vi "Parse State Queue__JKI_lib_State_Machine_ACBMOD.vi"(0 "State Queue":string, 7 "Error In":errorcluster) -> (4 "Remaining States":string, 6 "Current State":string, 8 "Arguments":string)   [LabVIEW 2015]
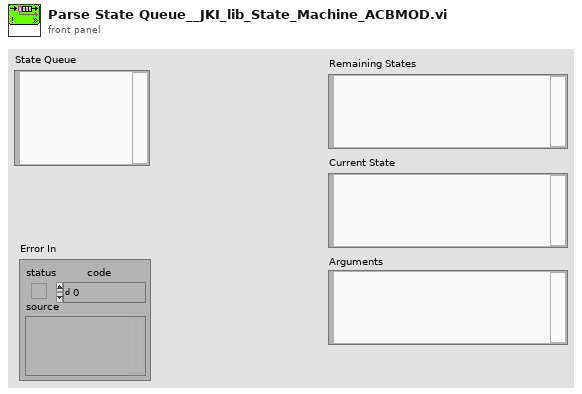
[diagram p1: front panel]
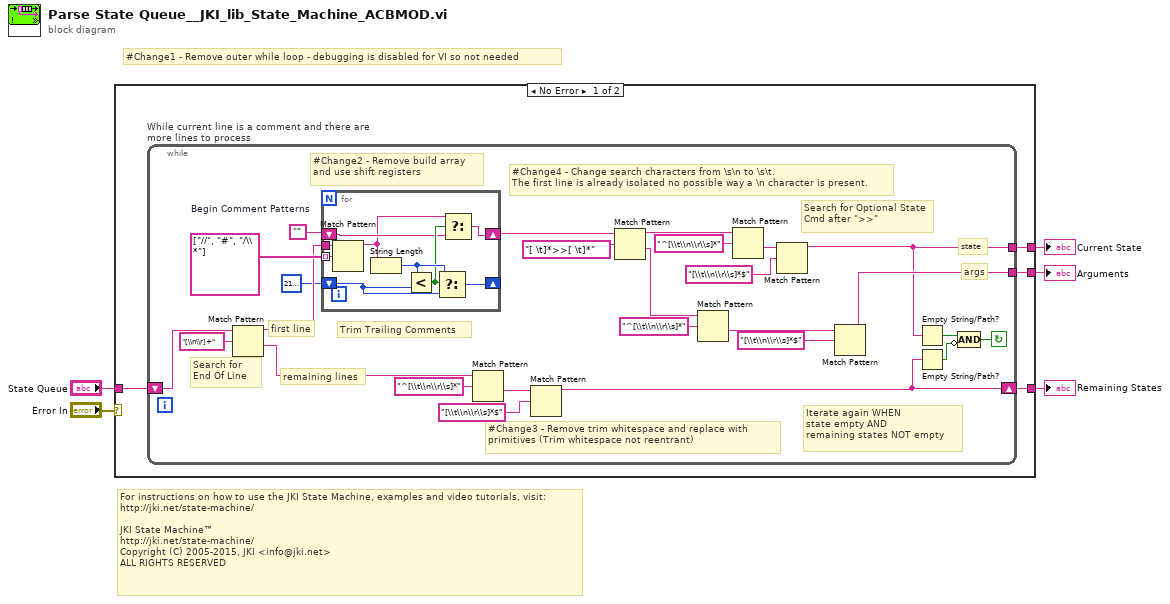
[diagram p0: block diagram]
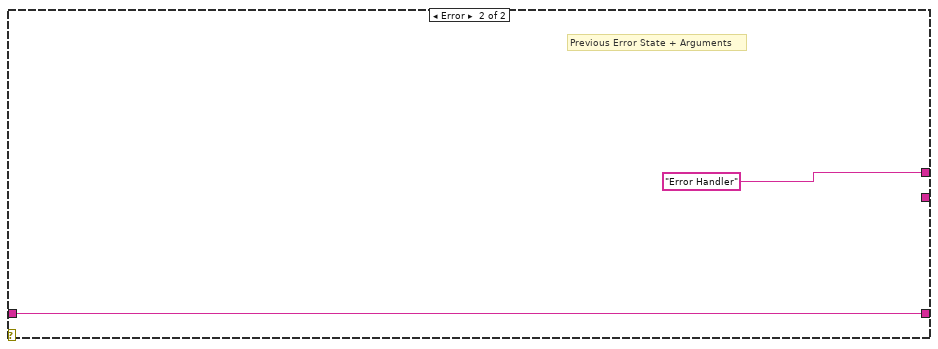
[diagram p2: hidden frame]
diagram:
  # "#Change1 - Remove outer while loop - debugging is disabled for VI so not needed"
  # "For instructions on how to use the JKI State Machine, examples and video tutorials, visit:\nhttp://jki.net/state-machine/\n\nJKI State Machine™\nhttp://jki.net/state-machine/\nCopyright (C) 2005-2015, JKI <info@jki.net>\nALL RIGHTS RESERVED"
  n1 = case shown="No Error" "Error In" {
    tunnel: [w6 w46] -> w5
    tunnel: [w9 "Error Handler"] -> w2
    tunnel: [w8 _] -> w1
    tunnel: "State Queue" -> [w7 w46]
    frame No Error {
      n2 = while "While current line is a comment and there are more lines to process" {
        tunnel: [w13] -> w9
        tunnel: [w21] -> w8
        shift-right: [w23] -> w6
        shift-left: w7 -> [w29]
        stop <- w31 continue-if-true
        w35 = string[] ["//", "#", "/\\*"]  # Begin Comment Patterns
        # "#Change4 - Change search characters from \\s\\n to \\s\\t.\nThe first line is already isolated no possible way a \\n character is present."
        # "#Change3 - Remove trim whitespace and replace with primitives (Trim whitespace not reentrant)"
        # "#Change2 - Remove build array and use shift registers"
        # "remaining lines"
        # "first line"
        # "Search for End Of Line"
        # "Iterate again WHEN\nstate empty AND\nremaining states NOT empty"
        # "args"
        # "state"
        # "Search for Optional State Cmd after \">>\""
        # "Trim Trailing Comments"
        n3 = Match Pattern(string=w29, regular expression="[\\n\\r]+") -> (before substring=w28:string, after substring=w24:string)  [unwired: 1 in, 2 out]
        n4 = for {
          tunnel: w28 -> [w44]
          tunnel: w35 -> [w43] mode=indexing
          shift-right: [w40] -> _
          shift-left: 2147483647 ("length") -> [w41]
          shift-right: [w38] -> w16
          shift-left: "" -> [w37]
          n5 = Match Pattern(string=w44, regular expression=w43) -> (before substring=w36:string)  [unwired: 1 in, 3 out]
          n6 = String Length(string=w36) -> (length=w42:i32)
          n7 = Less?(x=w42, y=w41) -> (x < y?=w39:bool)
          n8 = Select(t=w42, s=w39, f=w41) -> (s? t:f=w40:i32)
          n9 = Select(t=w36, s=w39, f=w37) -> (s? t:f=w38:string)
        }
        n10 = Match Pattern(string=w24, regular expression="^[\\t\\n\\r\\s]*") -> (after substring=w26:string)  [unwired: 1 in, 3 out]
        n11 = Match Pattern(string=w26, regular expression="[\\t\\n\\r\\s]*$") -> (before substring=w23:string)  [unwired: 1 in, 3 out]
        n12 = Match Pattern(string=w16, regular expression="[ \t]*>>[ \t]*") -> (before substring=w19:string, after substring=w11:string)  [unwired: 1 in, 2 out]
        n13 = Match Pattern(string=w11, regular expression="^[\\t\\n\\r\\s]*") -> (after substring=w10:string)  [unwired: 1 in, 3 out]
        n14 = Match Pattern(string=w19, regular expression="^[\\t\\n\\r\\s]*") -> (after substring=w14:string)  [unwired: 1 in, 3 out]
        n15 = Match Pattern(string=w14, regular expression="[\\t\\n\\r\\s]*$") -> (before substring=w13:string)  [unwired: 1 in, 3 out]
        n16 = Match Pattern(string=w10, regular expression="[\\t\\n\\r\\s]*$") -> (before substring=w21:string)  [unwired: 1 in, 3 out]
        n17 = Empty String/Path?(string/path=w13) -> (empty?=w33:bool)
        n18 = Empty String/Path?(string/path=w23) -> (empty?=w32:bool)
        n19 = Compound Arithmetic op=AND(w33, invert w32) -> (w31:bool)
      }
    }
    frame Error {
      # "Previous Error State + Arguments"
    }
  }
  "Remaining States" <- w5
  "Arguments" <- w1
  "Current State" <- w2
